vi "ReadWhileLoop.vi"(1 "reference":refnum<vi>) -> (0 "WhileLoop":T5)   [LabVIEW 2013]
uses:
  <vilib>/Utility/miscctls.llb/LVBoundsTypeDef.ctl
  <vilib>/Utility/miscctls.llb/LVPositionTypeDef.ctl
  <vilib>/Utility/miscctls.llb/LVRectTypeDef.ctl
  <vilib>/Utility/miscctls.llb/LVBreakpointStatusEnum.ctl
panel:
  out "error out 33":errorcluster
  out "error out 32":errorcluster
  out "error out 31":errorcluster
  out "error out 30":errorcluster
  out "error out 29":errorcluster
  out "error out 28":errorcluster
  out "error out 27":errorcluster
  out "error out 26":errorcluster
  out "error out 25":errorcluster
  out "error out 24":errorcluster
  out "error out 23":errorcluster
  out "error out 22":errorcluster
  out "error out 21":errorcluster
  out "error out 20":errorcluster
  out "error out 19":errorcluster
  out "error out 18":errorcluster
  out "error out 17":errorcluster
  out "error out 16":errorcluster
  out "error out 15":errorcluster
  out "error out 14":errorcluster
  out "error out 13":errorcluster
  out "error out 12":errorcluster
  out "error out 11":errorcluster
  out "error out 10":errorcluster
  out "error out 9":errorcluster
  out "error out 8":errorcluster
  out "error out 7":errorcluster
  out "error out 6":errorcluster
  out "error out 5":errorcluster
  out "error out 4":errorcluster
  out "error out 3":errorcluster
  out "error out 2":errorcluster
  out "error out":errorcluster
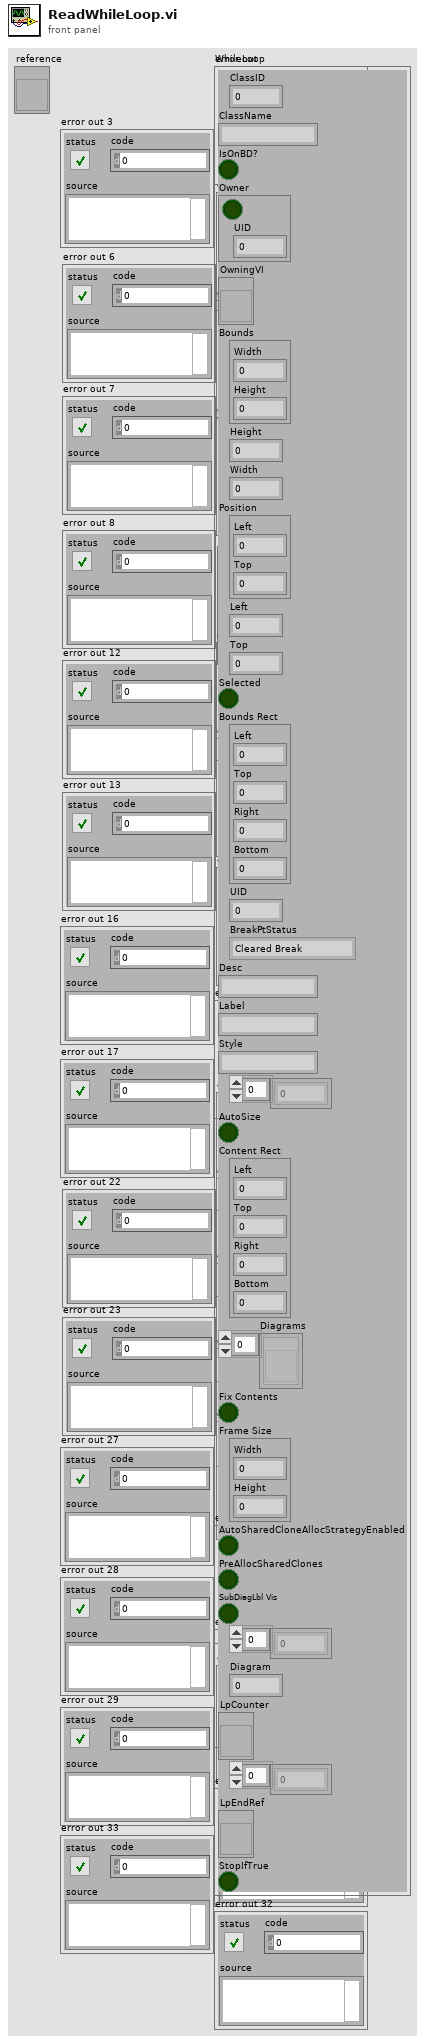
[diagram p1: front panel]
types:
  T1 = typedef "LVBoundsTypeDef.ctl" = cluster{"Width":u32, "Height":u32}
  T2 = typedef "LVPositionTypeDef.ctl" = cluster{"Left":i32, "Top":i32}
  T3 = typedef "LVRectTypeDef.ctl" = cluster{"Left":i16, "Top":i16, "Right":i16, "Bottom":i16}
  T4 = typedef "LVBreakpointStatusEnum.ctl" = enum8{"Cleared Break", "Enabled Break", "Disabled Break"}
  T5 = cluster{"ClassID":u32, "ClassName":string, "IsOnBD?":bool, "Owner":cluster{bool, "UID":i32}, "OwningVI":refnum<vi>, "Bounds":T1, "Height":u32, "Width":u32, "Position":T2, "Left":i32, "Top":i32, "Selected":bool, "Bounds Rect":T3, "UID":i32, "BreakPtStatus":T4, "Desc":string, "Label":string, "Style":string, "Terms[]":i32[], "AutoSize":bool, "Content Rect":T3, "Diagrams":refnum<vi>[], "Fix Contents":bool, "Frame Size":T1, "AutoSharedCloneAllocStrategyEnabled":bool, "PreAllocSharedClones":bool, "SubDiagLbl Vis":bool, "Tunnels[]":i32[], "Diagram":i32, "LpCounter":refnum<vi>, "ShiftRegs[]":i32[], "LpEndRef":refnum<vi>, "StopIfTrue":bool}
  T6 = cluster{"ClassID":u32, "ClassName":string, "IsOnBD?":bool, "Cluster":cluster{bool, "UID":i32}, "OwningVI":refnum<vi>, "Bounds":T1, "Height":u32, "Width":u32, "Position":T2, "Left":i32, "Top":i32, "Selected":bool, "Bounds Rect":T3, "UID":i32, "BreakPtStatus":T4, "Desc":string, "Text":string, "Style":string, i32[], "AutoSize":bool, "Content Rect":T3, "Diagrams":refnum<vi>[], "Fix Contents":bool, "Frame Size":T1, "AutoSharedCloneAllocStrategyEnabled":bool, "PreAllocSharedClones":bool, "SubDiagLbl Vis":bool, i32[], "UID":i32, "LpCounter":refnum<vi>, i32[], "LpEndRef":refnum<vi>, "StopIfTrue":bool}
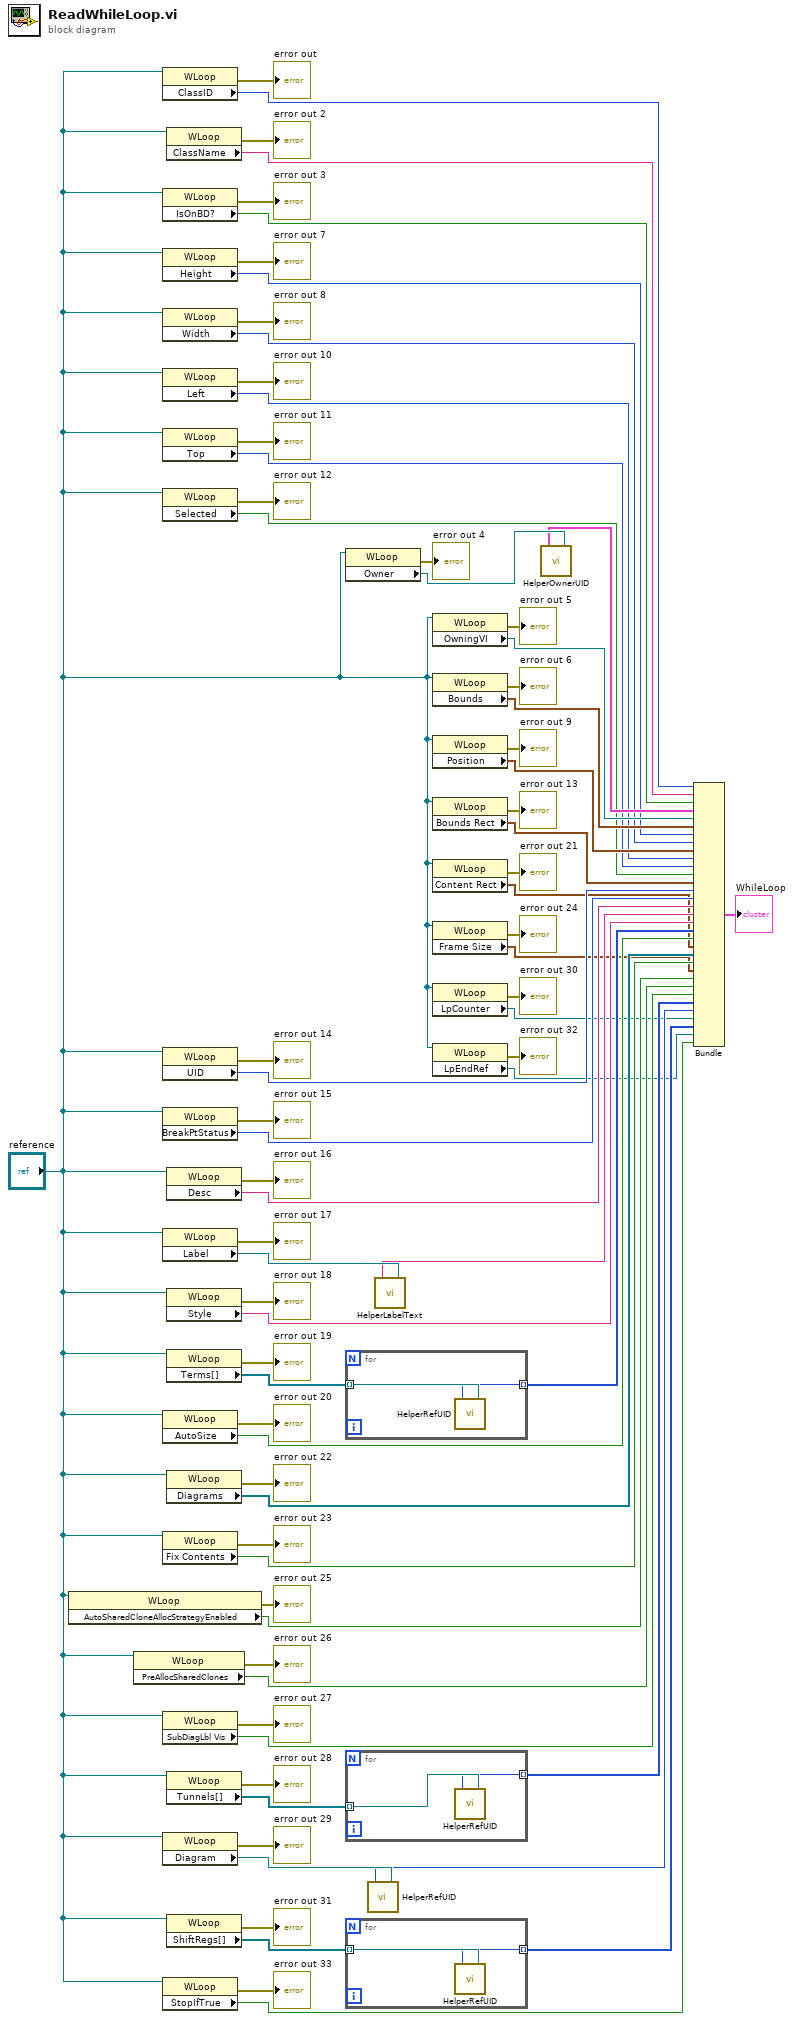
[diagram p0: block diagram]
diagram:
  n1 = property class="WLoop"(reference="reference") -> (error out=→"error out 25":errorcluster, "AutoSharedCloneAllocStrategyEnabled"=w21:bool)  [unwired: 1 in, 1 out]
  n2 = property class="WLoop"(reference="reference") -> (error out=→"error out 26":errorcluster, "PreAllocSharedClones"=w19:bool)  [unwired: 1 in, 1 out]
  n3 = property class="WLoop"(reference="reference") -> (error out=→"error out":errorcluster, "ClassID"=w72:u32)  [unwired: 1 in, 1 out]
  n4 = property class="WLoop"(reference="reference") -> (error out=→"error out 3":errorcluster, "IsOnBD?"=w68:bool)  [unwired: 1 in, 1 out]
  n5 = property class="WLoop"(reference="reference") -> (error out=→"error out 7":errorcluster, "Height"=w59:u32)  [unwired: 1 in, 1 out]
  n6 = property class="WLoop"(reference="reference") -> (error out=→"error out 8":errorcluster, "Width"=w57:u32)  [unwired: 1 in, 1 out]
  n7 = property class="WLoop"(reference="reference") -> (error out=→"error out 10":errorcluster, "Left"=w53:i32)  [unwired: 1 in, 1 out]
  n8 = property class="WLoop"(reference="reference") -> (error out=→"error out 11":errorcluster, "Top"=w51:i32)  [unwired: 1 in, 1 out]
  n9 = property class="WLoop"(reference="reference") -> (error out=→"error out 12":errorcluster, "Selected"=w49:bool)  [unwired: 1 in, 1 out]
  n10 = property class="WLoop"(reference="reference") -> (error out=→"error out 14":errorcluster, "UID"=w45:i32)  [unwired: 1 in, 1 out]
  n11 = property class="WLoop"(reference="reference") -> (error out=→"error out 15":errorcluster, "BreakPtStatus"=w43:T4)  [unwired: 1 in, 1 out]
  n12 = property class="WLoop"(reference="reference") -> (error out=→"error out 17":errorcluster, "Label"=w39:refnum<vi>)  [unwired: 1 in, 1 out]
  n13 = property class="WLoop"(reference="reference") -> (error out=→"error out 20":errorcluster, "AutoSize"=w31:bool)  [unwired: 1 in, 1 out]
  n14 = property class="WLoop"(reference="reference") -> (error out=→"error out 23":errorcluster, "Fix Contents"=w25:bool)  [unwired: 1 in, 1 out]
  n15 = property class="WLoop"(reference="reference") -> (error out=→"error out 27":errorcluster, "SubDiagLbl Vis"=w17:bool)  [unwired: 1 in, 1 out]
  n16 = property class="WLoop"(reference="reference") -> (error out=→"error out 29":errorcluster, "Diagram"=w12:refnum<vi>)  [unwired: 1 in, 1 out]
  n17 = property class="WLoop"(reference="reference") -> (error out=→"error out 33":errorcluster, "StopIfTrue"=w2:bool)  [unwired: 1 in, 1 out]
  n18 = property class="WLoop"(reference="reference") -> (error out=→"error out 2":errorcluster, "ClassName"=w70:string)  [unwired: 1 in, 1 out]
  n19 = property class="WLoop"(reference="reference") -> (error out=→"error out 16":errorcluster, "Desc"=w41:string)  [unwired: 1 in, 1 out]
  n20 = property class="WLoop"(reference="reference") -> (error out=→"error out 18":errorcluster, "Style"=w36:string)  [unwired: 1 in, 1 out]
  n21 = property class="WLoop"(reference="reference") -> (error out=→"error out 19":errorcluster, "Terms[]"=w34:refnum<vi>[])  [unwired: 1 in, 1 out]
  n22 = property class="WLoop"(reference="reference") -> (error out=→"error out 22":errorcluster, "Diagrams"=w27:refnum<vi>[])  [unwired: 1 in, 1 out]
  n23 = property class="WLoop"(reference="reference") -> (error out=→"error out 28":errorcluster, "Tunnels[]"=w15:refnum<vi>[])  [unwired: 1 in, 1 out]
  n24 = property class="WLoop"(reference="reference") -> (error out=→"error out 31":errorcluster, "ShiftRegs[]"=w7:refnum<vi>[])  [unwired: 1 in, 1 out]
  n25 = property class="WLoop"(reference="reference") -> (error out=→"error out 4":errorcluster, "Owner"=w66:refnum<vi>)  [unwired: 1 in, 1 out]
  n26 = for {
    tunnel: w34 -> [w76] mode=indexing
    tunnel: [w75] -> w33 mode=indexing
    n27 = call "HelperRefUID.vi"("Text in"=w76) -> ("UID"=w75:i32)
  }
  n28 = for {
    tunnel: w15 -> [w78] mode=indexing
    tunnel: [w77] -> w14 mode=indexing
    n29 = call "HelperRefUID.vi"("Text in"=w78) -> ("UID"=w77:i32)
  }
  n30 = for {
    tunnel: w7 -> [w80] mode=indexing
    tunnel: [w79] -> w6 mode=indexing
    n31 = call "HelperRefUID.vi"("Text in"=w80) -> ("UID"=w79:i32)
  }
  n32 = call "HelperRefUID.vi"("Text in"=w12) -> ("UID"=w11:i32)
  n33 = call "HelperLabelText.vi"("Text in"=w39) -> ("Text"=w38:string)
  n34 = property class="WLoop"(reference="reference") -> (error out=→"error out 5":errorcluster, "OwningVI"=w63:refnum<vi>)  [unwired: 1 in, 1 out]
  n35 = property class="WLoop"(reference="reference") -> (error out=→"error out 6":errorcluster, "Bounds"=w61:T1)  [unwired: 1 in, 1 out]
  n36 = property class="WLoop"(reference="reference") -> (error out=→"error out 9":errorcluster, "Position"=w55:T2)  [unwired: 1 in, 1 out]
  n37 = property class="WLoop"(reference="reference") -> (error out=→"error out 13":errorcluster, "Bounds Rect"=w47:T3)  [unwired: 1 in, 1 out]
  n38 = property class="WLoop"(reference="reference") -> (error out=→"error out 21":errorcluster, "Content Rect"=w29:T3)  [unwired: 1 in, 1 out]
  n39 = property class="WLoop"(reference="reference") -> (error out=→"error out 24":errorcluster, "Frame Size"=w23:T1)  [unwired: 1 in, 1 out]
  n40 = property class="WLoop"(reference="reference") -> (error out=→"error out 30":errorcluster, "LpCounter"=w9:refnum<vi>)  [unwired: 1 in, 1 out]
  n41 = property class="WLoop"(reference="reference") -> (error out=→"error out 32":errorcluster, "LpEndRef"=w4:refnum<vi>)  [unwired: 1 in, 1 out]
  n42 = call "HelperOwnerUID.vi"("Generic in"=w66) -> ("Cluster"=w65:cluster{bool, "UID":i32})
  n43 = Bundle("ClassID"=w72, "ClassName"=w70, "IsOnBD?"=w68, "Cluster"=w65, "OwningVI"=w63, "Bounds"=w61, "Height"=w59, "Width"=w57, "Position"=w55, "Left"=w53, "Top"=w51, "Selected"=w49, "Bounds Rect"=w47, "UID"=w45, "BreakPtStatus"=w43, "Desc"=w41, "Text"=w38, "Style"=w36, w33, "AutoSize"=w31, "Content Rect"=w29, "Diagrams"=w27, "Fix Contents"=w25, "Frame Size"=w23, "AutoSharedCloneAllocStrategyEnabled"=w21, "PreAllocSharedClones"=w19, "SubDiagLbl Vis"=w17, w14, "UID"=w11, "LpCounter"=w9, w6, "LpEndRef"=w4, "StopIfTrue"=w2) -> (→"WhileLoop":T6)  [unwired: 1 in]
